vi "Read configuration.vi"(7 "force loading?":bool=TRUE, 8 "error in (no error)":errorcluster, 11 "BMC in":refnum<class "BMC.lvclass">) -> (0 "error out":errorcluster, 3 "BMC out":refnum<class "BMC.lvclass">)   [LabVIEW 2012, in "BMC.lvclass"]
doc: "Reads the XML-based configuration file and populates the configuration cluster accordingly. Configuration file name is <component ID>.xml."
uses:
  BMC.lvclass
  Murmex/LabVIEW/Murmex/Murmex/Murmex.lvclass
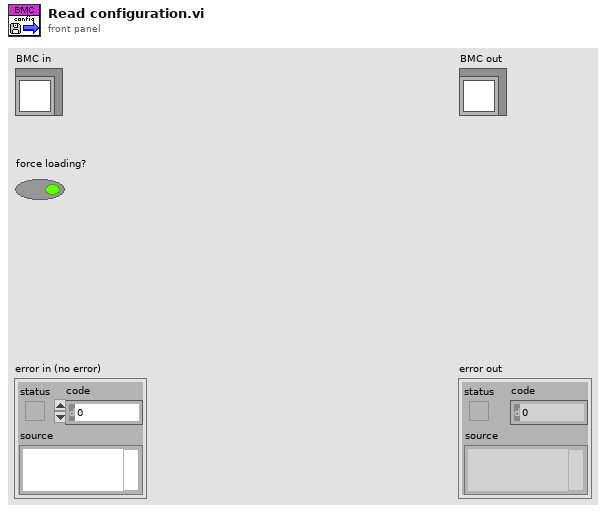
[diagram p1: front panel]
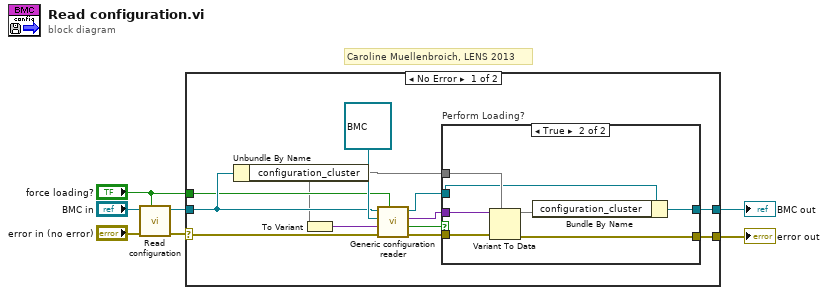
[diagram p0: block diagram]
diagram:
  # "Caroline Muellenbroich, LENS 2013"
  n1 = call-parent "Read configuration.vi"("force loading?"="force loading?", "error in (no error)"="error in (no error)", "Murmex in"="BMC in") -> ("error out"=w5:errorcluster, "Murmex out"=w4:refnum<class "BMC.lvclass">)  [unwired: 7 in]
  n2 = case shown="No Error" w5 {
    selector: w5 -> [w19 w29]
    tunnel: w4 -> [w16 w30]
    tunnel: "force loading?" -> [w15 _]
    tunnel: [w12 w29] -> w2
    tunnel: [w9 w30] -> w1
    frame No Error {
      n3 = Unbundle By Name(w16) -> ("configuration_cluster"=w11)
      n4 = To Variant(anything=w11) -> (Variant=w18:variant)
      n5 = call "Generic configuration reader.vi"("force loading?"=w15, "error in (no error)"=w19, "configuration cluster variant"=w18, "inheritance level"=refnum<class "BMC.lvclass"> refnum ("BMC"), "Murmex in"=w16) -> ("error out"=w13:errorcluster, "loaded?"=w14:bool, "configuration data (variant)"=w8:variant, "Murmex out"=w10:refnum<class "BMC.lvclass">)  [unwired: 3 in]
      n6 = case "Perform Loading?" shown="True" w14 {
        tunnel: w13 -> [w20 w28]
        tunnel: [w20 w27] -> w12
        tunnel: w11 -> [_ w26]
        tunnel: w10 -> [w21 w24]
        tunnel: [w21 w23] -> w9
        tunnel: w8 -> [_ w22]
        frame False {
        }
        frame True {
          n7 = Variant To Data(error in=w28, type=w26, Variant=w22) -> (data=w25, error out=w27:errorcluster)
          n8 = Bundle By Name(cluster=w24, "configuration_cluster"=w25) -> (w23:refnum<class "BMC.lvclass">)
        }
      }
    }
    frame Error {
    }
  }
  "error out" <- w2
  "BMC out" <- w1
